vi "Untitled 9.vi"() -> ()   [LabVIEW 2017]
panel:
  in  "string":string="asdasdasdasdasdasd"
  out "offset after match":i32
  out "substring after match":string
  out "substring before match":string
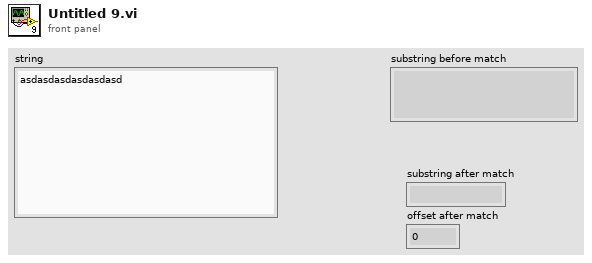
[diagram p1: front panel]
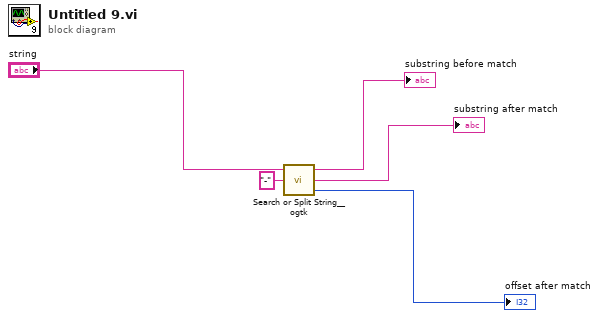
[diagram p0: block diagram]
diagram:
  n1 = call <userlib>:"Search or Split String__ogtk.vi"("search string/char (-)"="-", "string"="string") -> ("offset after match"=→"offset after match":i32, "substring after match"=→"substring after match":string, "substring before match"=→"substring before match":string)  [unwired: 1 in]
